vi "AccountDatabase.vi"(0 "Account_Details":T1=[{"Card Number"=11.0, "Card Holder Name"="Tom", "Valid Upto"=2050.0}, {"Card Number"=12.0, "Card Holder Name"="Jerry", "Valid Upto"=2024.0}, {"Card Number"=110.0, "Card Holder Name"="Jerry", "Valid Upto"=2050.0}], 1 "OK Button":bool, 5 "Search Option":T5(ring), 7 "Card Holder Name":string, 9 "Card Number":dbl, 11 "Valid Upto":dbl) -> (4 "Card Holder Name Search Result":T4, 6 "Card Number Search Result":T3, 8 "Valid Upto Search Result":T2, 10 "Search Time(ms)":dbl)   [LabVIEW 2020]
doc: "This VI contains a database of account details of many peoples and to search the credentials of many people based on card number, account holder name and validity of the card"
uses:
  Typedefs/Card holder name search result.ctl
  Typedefs/Card Validity search result.ctl
  Typedefs/AccountDetails.ctl
panel:
  # "Database"
  # "Search Box"
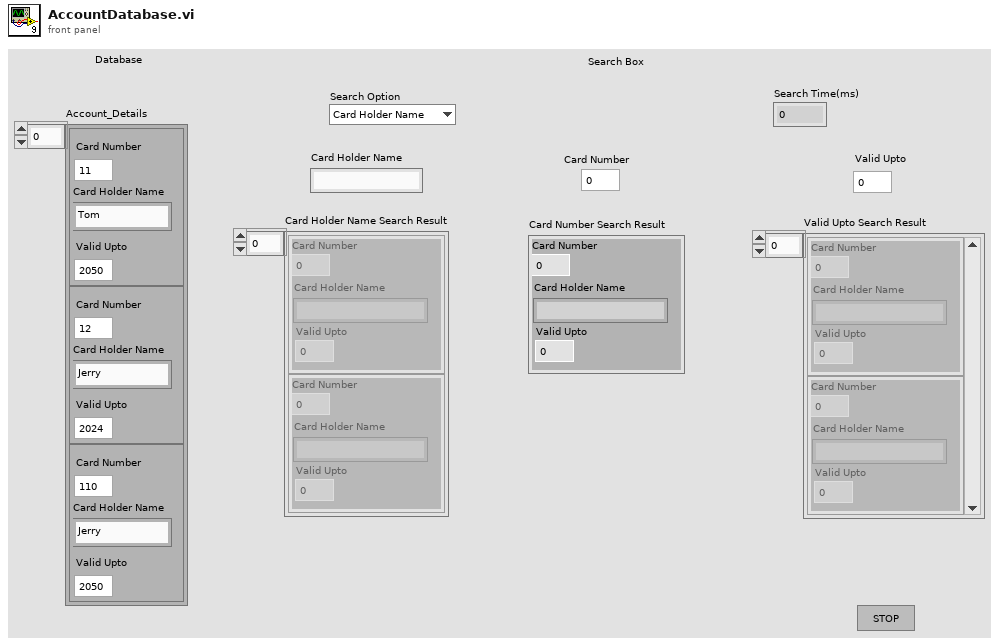
[diagram p1: front panel]
types:
  T1 = typedef "AccountDetails.ctl" = cluster{"Card Number":dbl, "Card Holder Name":string, "Valid Upto":dbl}[]
  T2 = typedef "Card Validity search result.ctl" = cluster{"Card Number":dbl, "Card Holder Name":string, "Valid Upto":dbl}[]
  T3 = cluster{"Card Number":dbl, "Card Holder Name":string, "Valid Upto":dbl}
  T4 = typedef "Card holder name search result.ctl" = cluster{"Card Number":dbl, "Card Holder Name":string, "Valid Upto":dbl}[]
  T5 = enum16{"Card Holder Name", "Card Number", "Valid Upto"}
  T6 = cluster{"Card Number":dbl, "Card Holder Name":string, "Valid Upto":dbl}[]
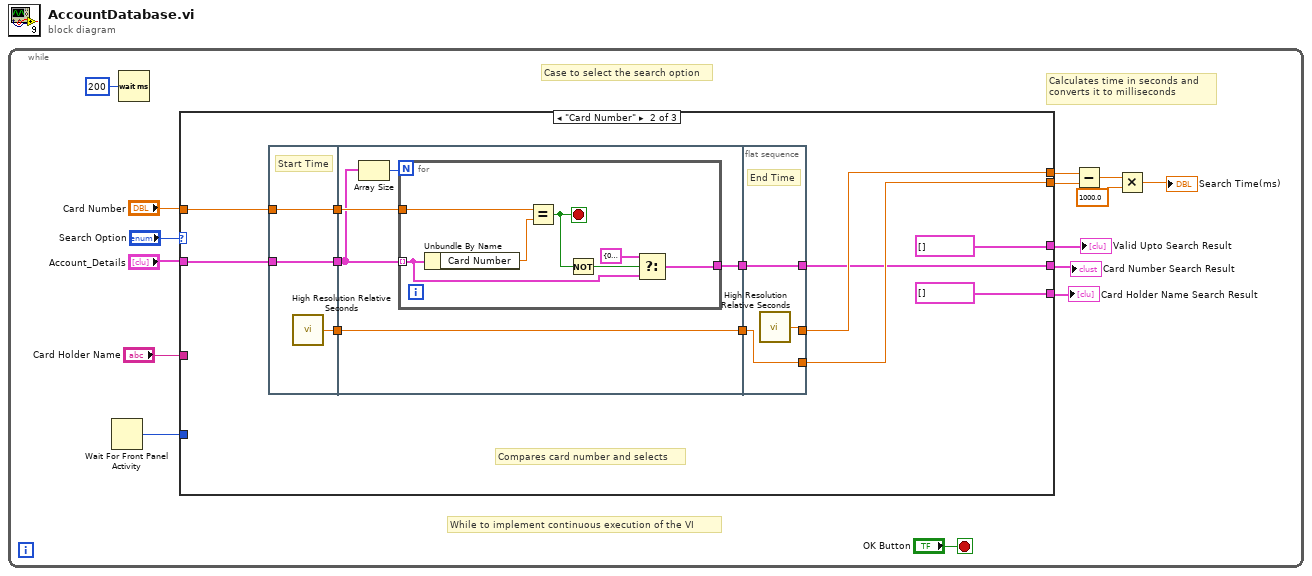
[diagram p0: block diagram]
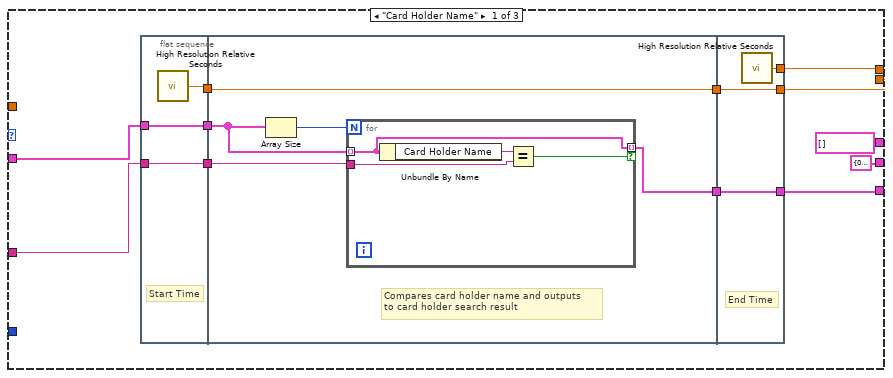
[diagram p2: hidden frame]
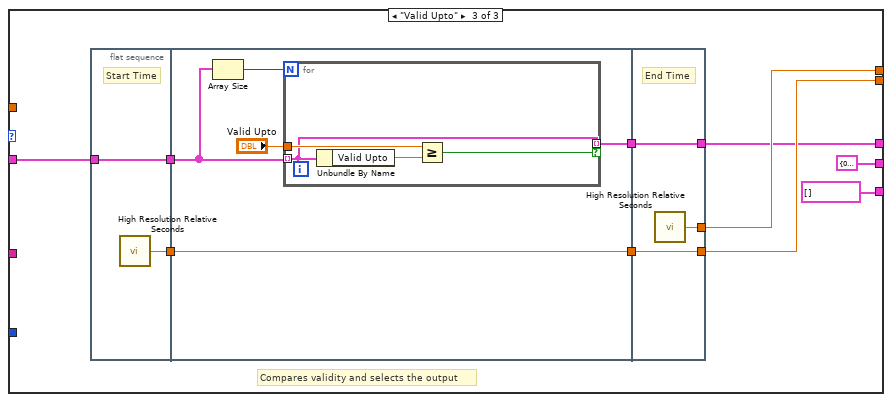
[diagram p3: hidden frame]
diagram:
  n1 = while {
    stop <- "OK Button" stop-if-true
    # "Calculates time in seconds and \nconverts it to milliseconds"
    # "While to implement continuous execution of the VI"
    # "Case to select the search option"
    n2 = Wait For Front Panel Activity() -> (0:w9:u32)  [unwired: 3 in]
    n3 = Wait (ms)(milliseconds to wait=u32 200) -> ()  [unwired: 1 out]
    n4 = case shown="\"Card Number\"" "Search Option" {
      tunnel: "Card Holder Name" -> [w26 _ _]
      tunnel: "Account_Details" -> [w27 w53 w82]
      tunnel: "Card Number" -> [_ w54 _]
      tunnel: w9 -> [_ _ _]
      tunnel: [w21 w47 w77] -> w6
      tunnel: [w20 w46 w76] -> w5
      tunnel: [T6 [] T6 [] w75] -> w3
      tunnel: [T3 {"Card Number"=0.0, "Card Holder Name"="", "Valid Upto"=0.0} ("Account_Details") w45 T3 {"Card Number"=0.0, "Card Holder Name"="", "Valid Upto"=0.0} ("Account_Details")] -> w2
      tunnel: [w18 T6 [] T6 []] -> w1
      frame "Card Holder Name" {
        n5 = flat-sequence {
          tunnel: w26 -> [w29]
          tunnel: w27 -> [w30]
          tunnel: [w30] -> w25
          tunnel: [w29] -> w24
          tunnel: [w28] -> w22
          tunnel: w25 -> [w34]
          tunnel: w24 -> [w33]
          tunnel: [w32] -> w23
          tunnel: w22 -> [w32]
          tunnel: [w31] -> w19
          tunnel: w23 -> [w41]
          tunnel: [w42] -> w21
          tunnel: [w41] -> w20
          tunnel: w19 -> [w40]
          tunnel: [w40] -> w18
          frame #0 {
            # "Start Time"
            n6 = call <vilib>:"High Resolution Relative Seconds.vi"() -> ("relative seconds"=w28:dbl)
          }
          frame #1 {
            # "Compares card holder name and outputs\nto card holder search result"
            n7 = Array Size(array=w34) -> (size(s)=w35:i32)
            n8 = for {
              N: w35 -> [_]
              tunnel: w34 -> [w36] mode=indexing
              tunnel: w33 -> [w38]
              tunnel: [w36] -> w31 mode=indexing if=w37
              n9 = Unbundle By Name(w36) -> ("Card Holder Name"=w39:string)
              n10 = Equal?(x=w39, y=w38) -> (x = y?=w37:bool)
            }
          }
          frame #2 {
            # "End Time"
            n11 = call <vilib>:"High Resolution Relative Seconds.vi"() -> ("relative seconds"=w42:dbl)
          }
        }
      }
      frame "Card Number" {
        # "Compares card number and selects"
        n12 = flat-sequence {
          tunnel: w53 -> [w56]
          tunnel: w54 -> [w57]
          tunnel: [w57] -> w51
          tunnel: [w56] -> w50
          tunnel: [w55] -> w48
          tunnel: [w59] -> w52
          tunnel: w51 -> [w62]
          tunnel: w50 -> [w60]
          tunnel: [w58] -> w49
          tunnel: w48 -> [w58]
          tunnel: [w72] -> w45
          tunnel: w52 -> [w72]
          tunnel: [w71] -> w47
          tunnel: w49 -> [w70]
          tunnel: [w70] -> w46
          frame #0 {
            # "Start Time"
            n13 = call <vilib>:"High Resolution Relative Seconds.vi"() -> ("relative seconds"=w55:dbl)
          }
          frame #1 {
            n14 = Array Size(array=w60) -> (size(s)=w61:i32)
            n15 = for {
              N: w61 -> [_]
              tunnel: w60 -> [w65] mode=indexing
              tunnel: w62 -> [w69]
              tunnel: [w63] -> w59
              stop <- w67 stop-if-true
              n16 = Unbundle By Name(w65) -> ("Card Number"=w68:dbl)
              n17 = Equal?(x=w69, y=w68) -> (x = y?=w67:bool)
              n18 = Not(x=w67) -> (.not. x?=w66:bool)
              n19 = Select(t=T3 {"Card Number"=0.0, "Card Holder Name"="", "Valid Upto"=0.0}, s=w66, f=w65) -> (s? t:f=w63:T3)
            }
          }
          frame #2 {
            # "End Time"
            n20 = call <vilib>:"High Resolution Relative Seconds.vi"() -> ("relative seconds"=w71:dbl)
          }
        }
      }
      frame "Valid Upto" {
        # "Compares validity and selects the output"
        n21 = flat-sequence {
          tunnel: w82 -> [w84]
          tunnel: [w84] -> w81
          tunnel: [w83] -> w78
          tunnel: w81 -> [w87]
          tunnel: [w86] -> w80
          tunnel: [w85] -> w79
          tunnel: w78 -> [w85]
          tunnel: [w96] -> w75
          tunnel: w80 -> [w96]
          tunnel: w79 -> [w94]
          tunnel: [w95] -> w77
          tunnel: [w94] -> w76
          frame #0 {
            # "Start Time"
            n22 = call <vilib>:"High Resolution Relative Seconds.vi"() -> ("relative seconds"=w83:dbl)
          }
          frame #1 {
            n23 = Array Size(array=w87) -> (size(s)=w88:i32)
            n24 = for {
              N: w88 -> [_]
              tunnel: "Valid Upto" -> [w93]
              tunnel: w87 -> [w90] mode=indexing
              tunnel: [w90] -> w86 mode=indexing if=w91
              n25 = Unbundle By Name(w90) -> ("Valid Upto"=w92:dbl)
              n26 = Greater Or Equal?(x=w93, y=w92) -> (x >= y?=w91:bool)
            }
          }
          frame #2 {
            # "End Time"
            n27 = call <vilib>:"High Resolution Relative Seconds.vi"() -> ("relative seconds"=w95:dbl)
          }
        }
      }
    }
    "Valid Upto Search Result" <- w3
    "Card Number Search Result" <- w2
    "Card Holder Name Search Result" <- w1
    n28 = Subtract(x=w6, y=w5) -> (x-y=w8:dbl)
    n29 = Multiply(x=w8, y=1000.0) -> (x*y=→"Search Time(ms)":dbl)
  }
